vi "Read Best Cost.vi"(8 "error in (no error)":errorcluster, 11 "State in":refnum<class "State.lvclass">) -> (0 "error out":errorcluster, 2 "Best Cost":u64, 3 "State out":refnum<class "State.lvclass">)   [LabVIEW 2019, in "23.lvlib" / "State.lvclass"]
uses:
  State.lvclass
  C:/Users/craig.walker/Documents/GitHub/lv2019-LRU-Cache/LRU Node/LRU Node.lvclass
  lv2019-LRU-Cache/LRU Node/LRU Node.lvclass/LRU Node.ctl
  State Value/State Value.lvclass
  lv2019-LRU-Cache/LRU Node/LRU Node.lvclass
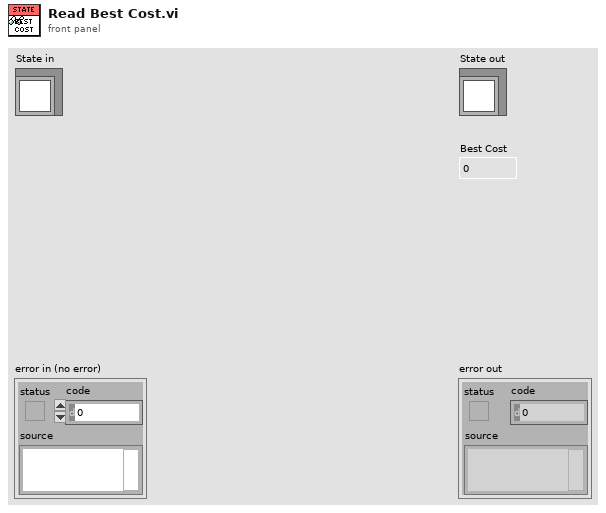
[diagram p1: front panel]
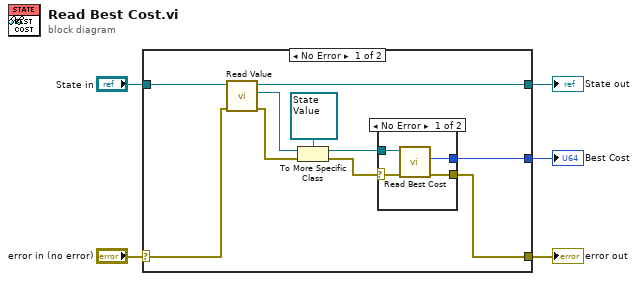
[diagram p0: block diagram]
diagram:
  n1 = case shown="No Error" "error in (no error)" {
    selector: "error in (no error)" -> [w7 w20]
    tunnel: [w6 w20] -> w4
    tunnel: [w15 w21] -> w2
    tunnel: "State in" -> [w10 w21]
    tunnel: [w11 _] -> w1
    frame No Error {
      n2 = call "Read Value.vi"("error in (no error)"=w7, "LRU Node in"=w10) -> ("error out"=w9:errorcluster, "Value"=w14:refnum<class>, "LRU Node out"=w15:refnum<class "State.lvclass">)  [unwired: 7 in]
      n3 = To More Specific Class(target class=refnum<class "State Value.lvclass"> refnum ("23.lvlib:State Value.lvclass"), reference=w14, error in=w9) -> (specific class reference=w12:refnum<class "State Value.lvclass">, error out=w8:errorcluster)
      n4 = case shown="No Error" w8 {
        selector: w8 -> [w17 _]
        tunnel: w12 -> [w19 _]
        tunnel: [w18 _] -> w11
        tunnel: [w16 _] -> w6
        frame No Error {
          n5 = call-dynamic "Read Best Cost.vi"("error in (no error)"=w17, "State Value in"=w19) -> ("error out"=w16:errorcluster, "Best Cost"=w18:u64)  [unwired: 7 in, 1 out]
        }
        frame Error {
        }
      }
    }
    frame Error {
    }
  }
  "error out" <- w4
  "State out" <- w2
  "Best Cost" <- w1
